vi "NI6071E.Disconnect.vi"(0 "i ref in":refnum<vi>, 5 "error in (no error)":errorcluster) -> (14 "i ref out":refnum<vi>, 19 "error out":errorcluster)   [LabVIEW 2014, in "NI6071E.lvlib"]
uses:
  NI6071E.lvlib
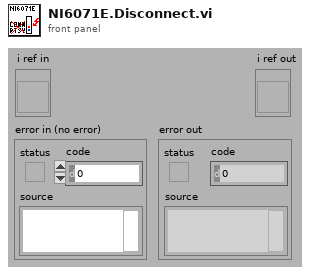
[diagram p1: front panel]
types:
  T1 = typedef "NI6071E.lvlib/NI6071E.i attribute.ctl" = cluster{"NI6071E Server":string, "Port":u16, "NI6071E Config":T2, "NI6071E Start":T3, "Waveforms":waveform(dbl)[], "RT Error":errorcluster, "NI6071E Read":T4, "connection ID":refnum<k5>, "DAQ Status":string, "device (1)":i16, "DAQ Status Service ID":i32}
  T2 = typedef "NI6071E.lvlib/NI6071EConfig.ctl" = cluster{"device (1)":i16, "channels (0)":tag[], "buffer size (1000 scans)":i32, "[number of buffers] (1)":i32, "measurement mode structure":cluster{"measurement mode":u16, "reserved":u32}, "input limits (no change)":cluster{"high limit (0.0)":sgl, "low limit (0.0)":sgl}[], "coupling & input config (no change:0)":cluster{"coupling (no change:0)":enum16{"no change", "DC", "AC", "GND", "internal ref."}, "input config (no change:0)":u16}[]}
  T3 = typedef "NI6071E.lvlib/NI6071EStart.ctl" = cluster{"scan rate (40000 scans/sec)":sgl, "trigger type (analog)":enum16{"no trigger", "analog", "digital A", "digital A & B", "scan clock gate"}, "edge or slope \n(rising)":enum16{"no change", "rising", "falling"}, "number of buffers to acquire (1)":i32, "analog chan (PFI0) & level (2.00)":cluster{"trigger channel (empty)":string, "level (0.0)":sgl}, "[additional trig params]":cluster{"hysteresis (0.0)":sgl, "coupling (no change:0)":enum16{"no change", "DC", "AC"}, "delay (0 sec)":sgl, "skip count (0)":i32, "time limit (0 sec)":sgl}}
  T4 = typedef "NI6071E.lvlib/NI6071ERead.ctl" = cluster{"time limit in sec (-1:auto calculate)":sgl, "number of scans to read (-1:all)":i32}
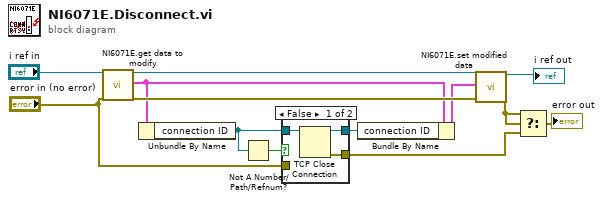
[diagram p0: block diagram]
diagram:
  n1 = call "NI6071E.get data to modify.vi"("i ref in"="i ref in", "error in (no error)"="error in (no error)") -> ("i ref out"=w11:refnum<vi>, "i attribute"=w5:T1, "error out"=w12:errorcluster)  [unwired: 14 in, 1 out]
  n2 = Unbundle By Name(w5) -> ("connection ID"=w3:refnum<k5>)
  n3 = Not A Number/Path/Refnum?(number/path/refnum=w3) -> (NaN/Path/Refnum?=w2:bool)
  n4 = case shown="False" w2 {
    tunnel: [w16 w18] -> w6
    tunnel: w3 -> [w15 w18]
    tunnel: [w14 w17] -> w4
    tunnel: "error in (no error)" -> [_ w17]
    frame False {
      n5 = TCP Close Connection(connection ID=w15) -> (connection ID out=w16:refnum<k5>, error out=w14:errorcluster)  [unwired: 2 in]
    }
    frame True {
    }
  }
  n6 = Bundle By Name(cluster=w5, "connection ID"=w6) -> (w7:T1)
  n7 = call "NI6071E.set modified data.vi"("i ref in"=w11, "i attribute"=w7, "error in (no error)"=w12) -> ("i ref out"=→"i ref out":refnum<vi>, "error out"=w9:errorcluster)  [unwired: 15 in]
  n8 = Select(t=w9, s=w9, f=w4) -> (s? t:f=→"error out":errorcluster)
